vi "Comb Filter.vi"(2 "n":i64, 3 "g":fxp<+/-,16,4>) -> ()   [LabVIEW 2016]
uses:
  <vilib>/rvi/Emulation/niFpgaSctlEmulationGetInTimedLoop.vi
  Global 1.vi
  <vilib>/rvi/Emulation/niFpgaProcessEmulError.vi
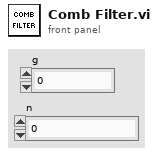
[diagram p1: front panel]
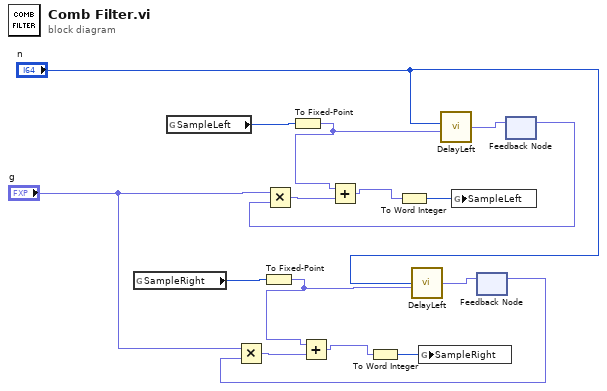
[diagram p0: block diagram]
diagram:
  n1 = global read "Global 1.vi" "SampleRight"() -> (w10:i16)
  n2 = global read "Global 1.vi" "SampleLeft"() -> (w15:i16)
  n3 = To Fixed-Point(number=w10) -> (fixed-point=w1:fxp<+/-,25,16>)  [unwired: 1 in]
  n4 = To Fixed-Point(number=w15) -> (fixed-point=w2:fxp<+/-,25,16>)  [unwired: 1 in]
  n5 = call "DelayLeft.vi"("sample in"=w1, "n"="n") -> ("SampleOut"=w9:fxp<+/-,25,16>)  [unwired: 2 in]
  n6 = call "DelayLeft.vi"("sample in"=w2, "n"="n") -> ("SampleOut"=w14:fxp<+/-,25,16>)  [unwired: 2 in]
  n7 = feedback #1() -> (w7:fxp<+/-,25,16>)  [unwired: 1 in]
  n8 = Multiply(x="g", y=w7) -> (x*y=w11:fxp<+/-,41,20>)
  n9 = Add(x=w1, y=w11) -> (x+y=w4:fxp<+/-,41,20>)
  n10 = To Word Integer(number=w4) -> (16bit integer=w8:i16)
  n11 = global write "Global 1.vi" "SampleRight"(w8) -> ()
  n12 = feedback-in #1(w9) -> ()
  n13 = feedback-in #2(w14) -> ()
  n14 = feedback #2() -> (w12:fxp<+/-,25,16>)  [unwired: 1 in]
  n15 = Multiply(x="g", y=w12) -> (x*y=w16:fxp<+/-,41,20>)
  n16 = Add(x=w2, y=w16) -> (x+y=w3:fxp<+/-,41,20>)
  n17 = To Word Integer(number=w3) -> (16bit integer=w13:i16)
  n18 = global write "Global 1.vi" "SampleLeft"(w13) -> ()
